vi "Write Pin.vi"(0 "Simulated Device in":refnum<class "Simulated Device.lvclass">, 5 "VISA resource name":refnum<visa-resource-name>, 7 "Pin":dbl, 9 "1/0":bool, 11 "error in (no error)":errorcluster) -> (4 "Simulated Device out":refnum<class "Simulated Device.lvclass">, 6 "VISA resource name 2":refnum<visa-resource-name>, 10 "Read":string, 15 "error out":errorcluster)   [LabVIEW 2020, in "Simulated Device.lvclass"]
uses:
  Simulated Device.lvclass
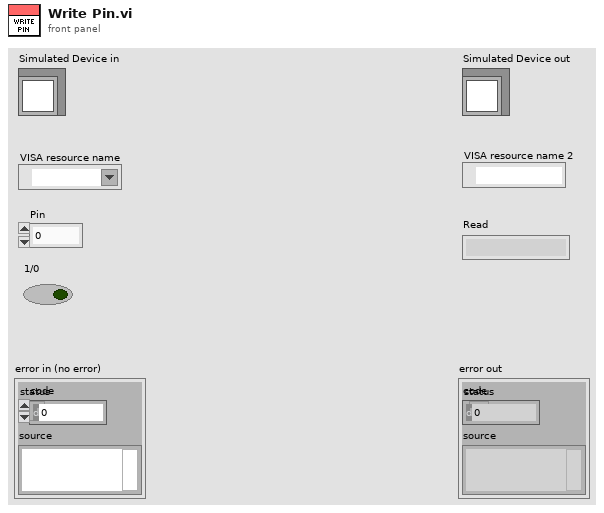
[diagram p1: front panel]
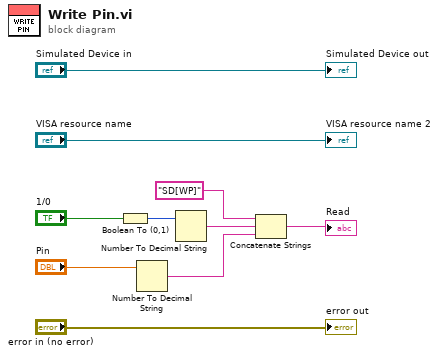
[diagram p0: block diagram]
diagram:
  n1 = Boolean To (0,1)(Boolean="1/0") -> (0, 1=w6:i16)
  n2 = Number To Decimal String(number="Pin") -> (decimal integer string=w2:string)  [unwired: 1 in]
  n3 = Number To Decimal String(number=w6) -> (decimal integer string=w5:string)  [unwired: 1 in]
  n4 = Concatenate Strings("SD[WP]" ("string"), w5, w2) -> (→"Read":string)
  "error out" <- "error in (no error)"
  "Simulated Device out" <- "Simulated Device in"
  "VISA resource name 2" <- "VISA resource name"
